vi "filtra per npsh.vi"(9 "Pto npsh":u8, 10 "Curva 1":string[][](array[string]), 11 "indici":T1) -> (2 "Cluster":cluster{"index":i32, "length":i32}, 3 "Boolean":bool)   [LabVIEW 2019]
uses:
  TypeDef/Indici.ctl
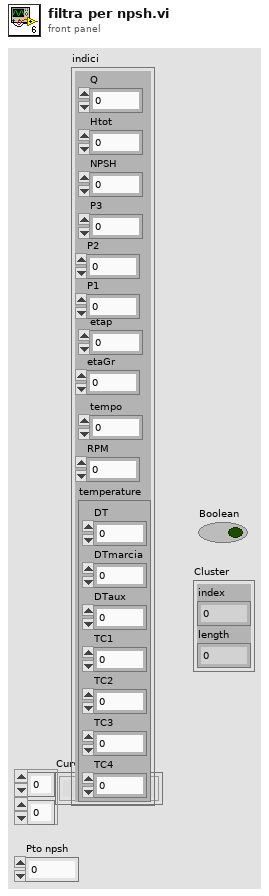
[diagram p1: front panel]
types:
  T1 = typedef "Indici.ctl" = cluster{"Q":i32, "Htot":i32, "NPSH":i32, "P3":i32, "etap":i32, "temperature":cluster{"DT":i32, "DTmarcia":i32, "DTaux":i32, "TC1":i32, "TC2":i32, "TC3":i32, "TC4":i32}, "tempo":i32, "P2":i32, "P1":i32, "etaGr":i32, "RPM":i32}
  T2 = cluster{"punto":i32, "cluster":cluster{"index":i32, "length":i32}}[]
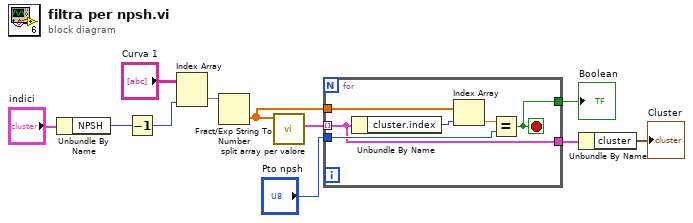
[diagram p0: block diagram]
diagram:
  n1 = Unbundle By Name("indici") -> ("NPSH"=w4:i32)
  n2 = Decrement(x=w4) -> (x-1=w10:i32)
  n3 = Index Array(array="Curva 1", index (col)=w10) -> (element=w5:string[])  [unwired: 1 in]
  n4 = Fract/Exp String To Number(string=w5) -> (number=w6:dbl[])  [unwired: 3 in, 1 out]
  n5 = call <userlib>:"split array per valore.vi"("Array"=w6) -> ("sorted array"=w2:T2)  [unwired: 10 in]
  n6 = for {
    tunnel: w2 -> [w14] mode=indexing
    tunnel: w6 -> [w17]
    tunnel: "Pto npsh" -> [w15]
    tunnel: [w14] -> w9
    tunnel: [w13] -> w8
    stop <- w13 stop-if-true
    n7 = Unbundle By Name(w14) -> ("cluster.index"=w12:i32)
    n8 = Index Array(array=w17, index=w12) -> (element=w16:dbl)
    n9 = Equal?(x=w16, y=w15) -> (x = y?=w13:bool)
  }
  "Boolean" <- w8
  n10 = Unbundle By Name(w9) -> ("cluster"=→"Cluster":cluster{"index":i32, "length":i32})
